vi "lumencor_off.vi"   [LabVIEW 2011]
uses:
  <vilib>/DAQmx/write.llb/DAQmx Write (Analog 1D DBL NChan 1Samp).vi
  <vilib>/DAQmx/miscellaneous.llb/DAQmx Fill In Error Info.vi
types:
  T1 = enum32{"Invalid", "Standard", "Closed", "Hidden", "Minimized", "Maximized"}
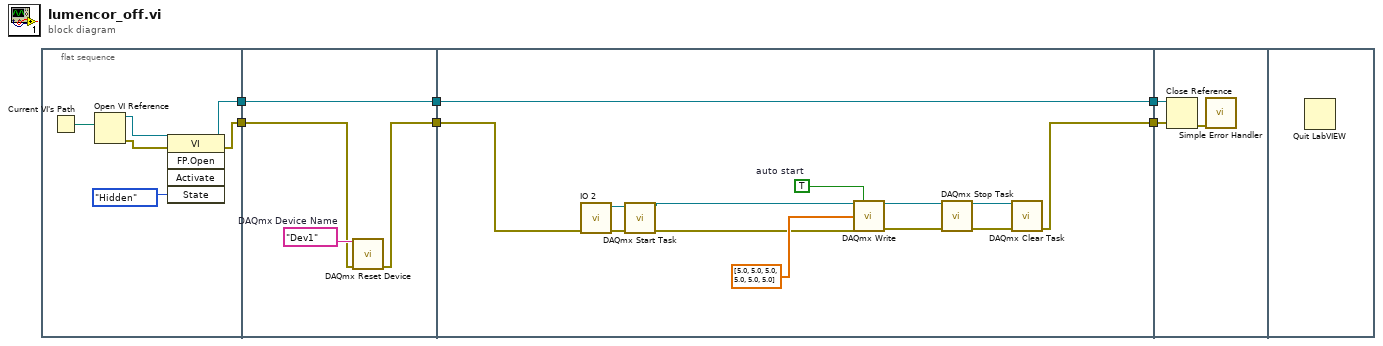
[diagram p0: block diagram]
diagram:
  n1 = flat-sequence {
    tunnel: [w8] -> w4
    tunnel: [w7] -> w2
    tunnel: w4 -> [w14]
    tunnel: [w13] -> w3
    tunnel: w2 -> [w16]
    tunnel: [w16] -> w1
    tunnel: [w17] -> w6
    tunnel: w3 -> [w18]
    tunnel: [w27] -> w5
    tunnel: w1 -> [w27]
    tunnel: w6 -> [w31]
    tunnel: w5 -> [w30]
    frame #0 {
      n2 = Current VI's Path() -> (path=w12:path)
      n3 = Open VI Reference(vi path=w12) -> (vi reference=w11:refnum<vi>, error out=w10:errorcluster)  [unwired: 5 in]
      n4 = invoke class="VI" method="FP.Open"(reference=w11, error in=w10, "State"=T1."Hidden") -> (reference out=w7:refnum<vi>, error out=w8:errorcluster)  [unwired: 2 in, 3 out]
    }
    frame #1 {
      w15 = tag "Dev1"  # DAQmx Device Name
      n5 = call <vilib>:"DAQmx Reset Device.vi"("device in"=w15, "error in"=w14) -> ("error out"=w13:errorcluster)  [unwired: 13 in]
    }
    frame #2 {
      w29 = TRUE  # auto start
      n6 = call "IO 2.vi"("error in"=w18) -> ("error out"=w19:errorcluster, "task out"=w22:refnum<k21>)  [unwired: 9 in]
      n7 = call <vilib>:"DAQmx Start Task.vi"("task/channels in"=w22, "error in"=w19) -> ("task out"=w21:refnum<k21>, "error out"=w20:errorcluster)  [unwired: 12 in]
      n8 = call-poly <vilib>:"DAQmx Write.vi"("task/channels in"=w21, "auto start"=w29, "data"=dbl[] [5.0, 5.0, 5.0, 5.0, 5.0, 5.0], "error in"=w20) -> ("task out"=w26:refnum<k21>, "error out"=w24:errorcluster)  [unwired: 10 out]
      n9 = call <vilib>:"DAQmx Stop Task.vi"("task/channels in"=w26, "error in"=w24) -> ("task out"=w25:refnum<k21>, "error out"=w23:errorcluster)  [unwired: 12 in]
      n10 = call <vilib>:"DAQmx Clear Task.vi"("task in"=w25, "error in"=w23) -> ("error out"=w17:errorcluster)  [unwired: 13 in]
    }
    frame #3 {
      n11 = Close Reference(reference=w30, error in (no error)=w31) -> (error out=w32:errorcluster)
      n12 = call <vilib>:"Simple Error Handler.vi"("error in (no error)"=w32) -> ()  [unwired: 4 in, 5 out]
    }
    frame #4 {
      n13 = Quit LabVIEW() -> ()  [unwired: 1 in]
    }
  }
